vi "(TestVI)DW7802 PWL Ramp Map Test.vi"() -> ()   [LabVIEW 2020]
uses:
  <vilib>/Analysis/1siggen.llb/Ramp Pattern by Samples.vi
  <vilib>/Analysis/NI_AALBase.lvlib
panel:
  out "추가된 배열 3":dbl[](array[numeric]) format="%.3f"
  out "추가된 배열 2":dbl[](array[numeric]) format="%.3f"
  out "웨이브폼 그래프":dbl[][](graph)
  out "추가된 배열":dbl[][](array[numeric])
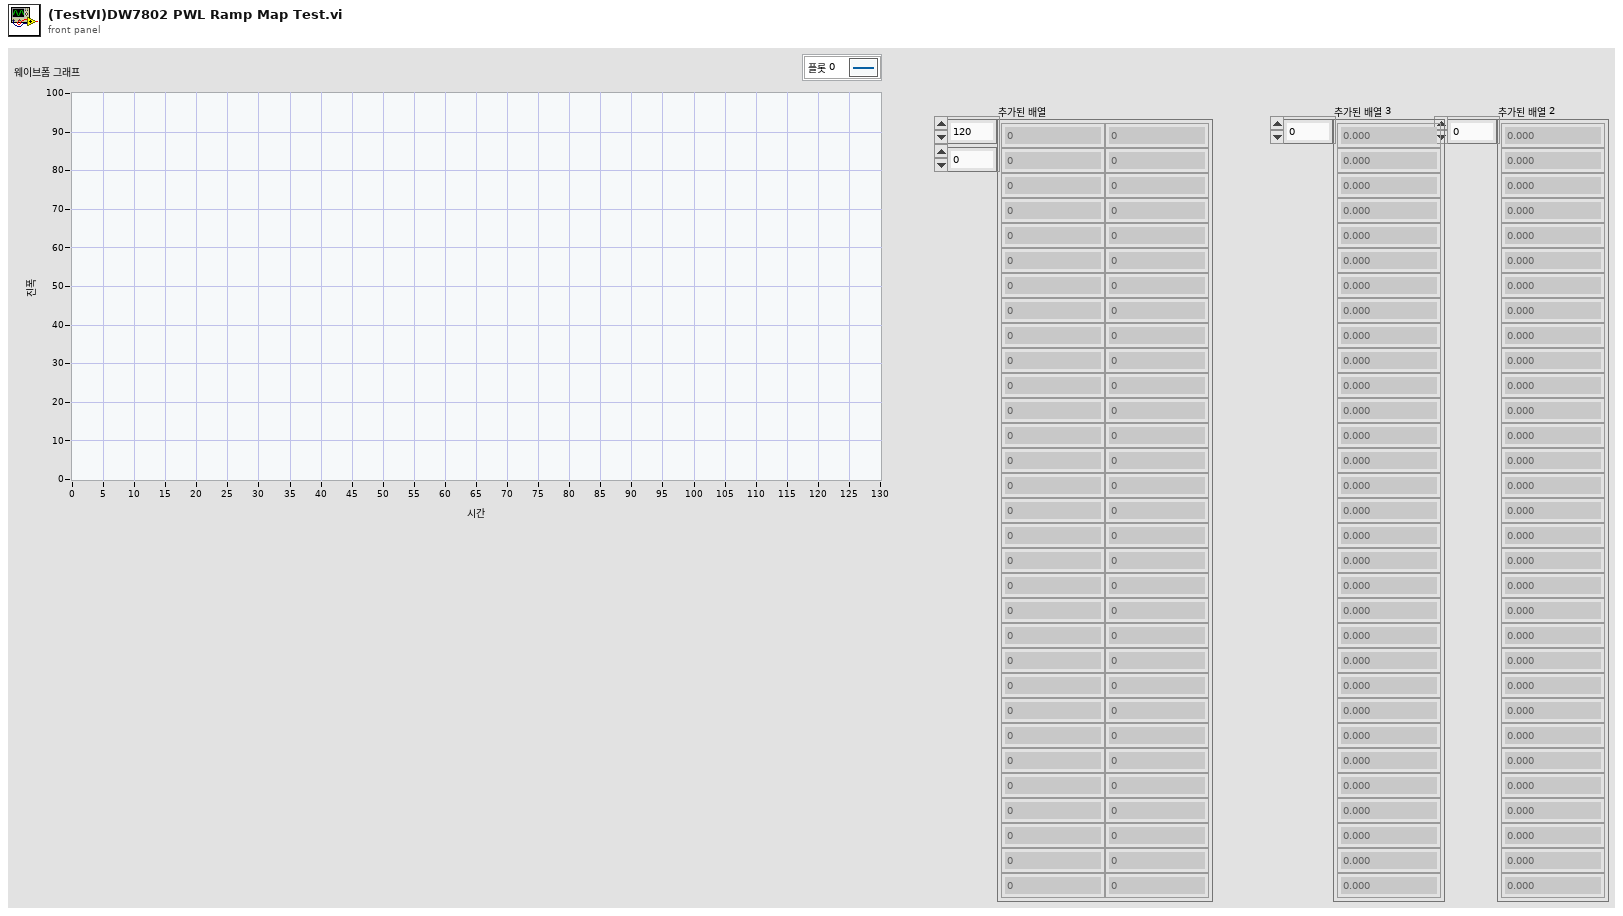
[diagram p1: front panel]
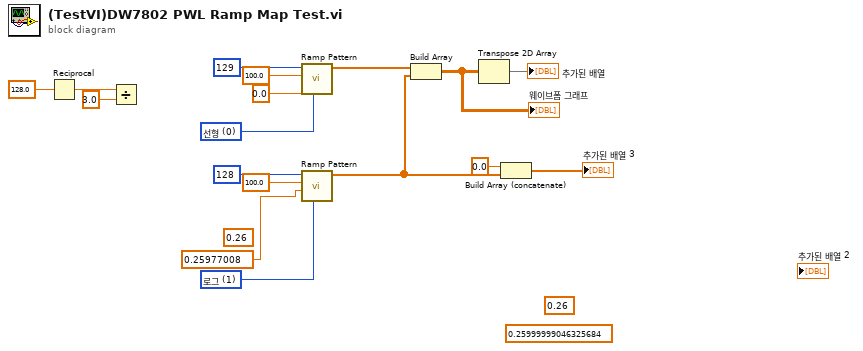
[diagram p0: block diagram]
diagram:
  (unwired) sgl 0.26
  (unwired) 0.26
  (unwired) 0.26 ("start")
  w8 = u16 1 items=["선형", "로그"] ("type")
  w14 = u16 0 items=["선형", "로그"] ("type")
  n1 = Reciprocal(x=128.0) -> (1/x=w3:dbl)
  n2 = Divide(x=w3, y=3.0) -> ()  [unwired: 1 out]
  n3 = call-poly <vilib>:"Ramp Pattern.vi"("type"=w14, "start"=0.0, "end"=100.0, "samples"=129) -> ("Ramp Pattern"=w12:dbl[])  [unwired: 6 in, 1 out]
  n4 = call-poly <vilib>:"Ramp Pattern.vi"("type"=w8, "start"=0.25977008, "end"=100.0, "samples"=128) -> ("Ramp Pattern"=w7:dbl[])  [unwired: 6 in, 1 out]
  n5 = Build Array(w12, w7) -> (w11:dbl[][])
  "웨이브폼 그래프" <- w11
  n6 = Transpose 2D Array(2D array=w11) -> (transposed array=→"추가된 배열":dbl[][])
  n7 = Build Array (concatenate)(0.0 ("원소"), w7) -> (→"추가된 배열 3":dbl[])
